vi "Open UDP connection.vi"(8 "error in (no error)":errorcluster) -> (0 "error out":errorcluster, 3 "connection ID":refnum<k16>)   [LabVIEW 2016]
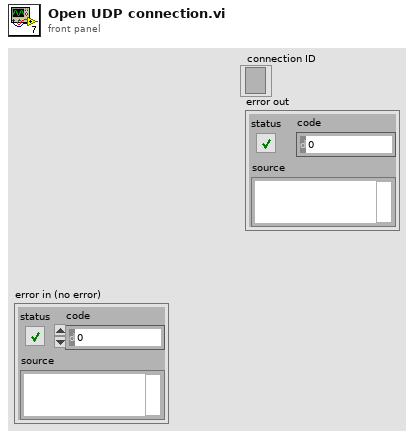
[diagram p1: front panel]
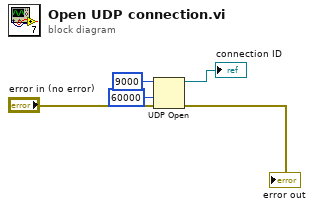
[diagram p0: block diagram]
diagram:
  n1 = UDP Open(8:"error in (no error)", 9:60000 ("timeout ms (25000)"), 11:u16 9000 ("port")) -> (port=→"connection ID":refnum<k16>, 0:→"error out":errorcluster)  [unwired: 2 in, 1 out]
